vi "Teleop.vi"(10 "Match Info":T1={"Autonomous Elapsed Seconds"=0.0, "TeleOp Elapsed Seconds"=0.0, "Disabled Elapsed Seconds"=0.0, "Visited Autonomous"=FALSE, "Visited TeleOp"=FALSE, "Visited Disabled"=FALSE, "Autonomous Settings"={"Autonomous Style"=enum."Independent", "VI Refnum"=refnum}}, 11 "Call Context":T2) -> ()   [LabVIEW 2014]
doc: "This VI is called for each TeleOp packet received from the DS where the robot is not disabled. It is often used to read from the joysticks and update I/O or to update setpoints for timed control loops. It should complete and return within 20 milliseconds or it may miss DS packets."
uses:
  <vilib>/Rock Robotics/WPI/DriverStation/WPI_DriverStationDerivedRobotMode.ctl
  <vilib>/Rock Robotics/WPI/DriverStation/WPI_DriverStationMatch Info.ctl
  <vilib>/Rock Robotics/WPI/Solenoid/WPI_SolenoidValue.ctl
  <vilib>/Rock Robotics/WPI/Relay/WPI_RelayValue.ctl
  <vilib>/Rock Robotics/WPI/RobotDrive/WPI_RobotDriveGetSetRefNum.vi
  <vilib>/Rock Robotics/WPI/Joystick/WPI_JoystickGetSetRefNum.vi
  Robot Global Data.vi
  <vilib>/Rock Robotics/WPI/Solenoid/WPI_SolenoidSetEnum.vi
panel:
  in  "last switch":bool
  in  "toggle on/off internal":bool=TRUE
  out "toggle on/off":bool=TRUE
  out "Sample Slider 0":dbl(slide) scale=0.0..5.0
  out "Sample Boolean 1":bool
  out "Sample Boolean 0":bool
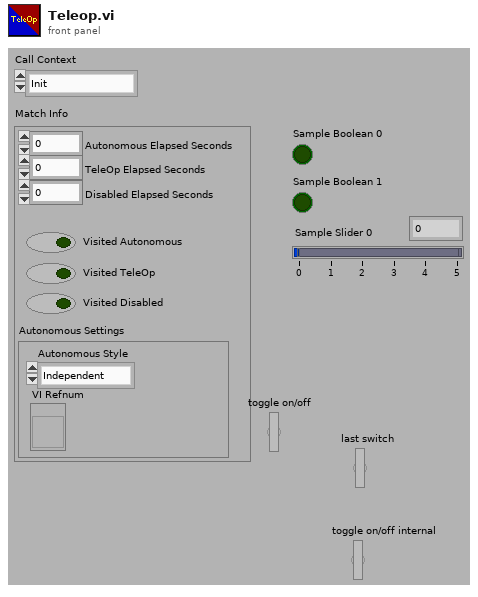
[diagram p1: front panel]
types:
  T1 = typedef "WPI_DriverStationMatch Info.ctl" = cluster{"Autonomous Elapsed Seconds":dbl, "TeleOp Elapsed Seconds":dbl, "Disabled Elapsed Seconds":dbl, "Visited Autonomous":bool, "Visited TeleOp":bool, "Visited Disabled":bool, "Autonomous Settings":cluster{"Autonomous Style":enum16{"Iterative", "Independent"}, "VI Refnum":refnum<vi>}}
  T2 = typedef "WPI_DriverStationDerivedRobotMode.ctl" = enum16{"Init", "Execute", "Stop"}
  T3 = typedef "WPI_RelayValue.ctl" = enum16{"Off", "On", "Forward", "Reverse"}
  T4 = typedef "WPI_SolenoidValue.ctl" = enum16{"Off", "On", "Forward", "Reverse"}
  T5 = typedef "WPI_RobotDriveDevRef.ctl" = cluster{"DevStatus":errorcluster, "Motors[]":T6[], "Square Inputs":bool, "Max Output":dbl}
  T6 = typedef "WPI_MotorControlDeviceRef.ctl" = cluster{"DeviceStatus":errorcluster, "Type":enum16{"PWM", "CAN"}, "PWM":cluster{"Digital Module":T7, "PWM Channel":T8, "DeadBand":T9}, "CAN":cluster{"Device Number":u8, "Control Mode":T10, "Semaphore":T11, "Max Vout":dbl}, "Invert":bool, "TransformRef":T12, "InvTransformRef":T12}
  T7 = typedef "FPGA_TypedefDigitalModule.ctl" = enum16{"Digital Module 1", "Digital Module 2"}
  T8 = typedef "FPGA_DIOPWMChannel.ctl" = enum8{"PWM 1", "PWM 2", "PWM 3", "PWM 4", "PWM 5", "PWM 6", "PWM 7", "PWM 8", "PWM 9", "PWM 10", "Invalid"}
  T9 = typedef "WPI_PWMDeadband.ctl" = cluster{"Name":string, "maxPositivePwm":i32, "minPositivePwm":i32, "centerPwm":i32, "maxNegativePwm":i32, "minNegativePwm":i32, "angularRange":u16}
  T10 = typedef "WPI_CANJaguar_ControlMode.ctl" = enum8{"Percent VBus", "Current", "Speed", "Position", "Voltage"}
  T11 = typedef "Semaphore RefNum" = refnum<k1>
  T12 = typedef "WPI_PWMTransform_ConPane.ctl" = refnum<vi>
  T13 = typedef "WPI_JoystickDevRef.ctl" = cluster{"Device":T14}
  T14 = typedef "WPI_JoystickDeviceEnum.ctl" = enum16{"USB 0", "USB 1", "USB 2", "USB 3", "USB 4", "USB 5"}
  T15 = typedef "WPI_RelayDevRef.ctl" = cluster{"DevStatus":errorcluster, "Relay Channel":T16, "Digital Module":T7, "Relay Direction":T17}
  T16 = typedef "FPGA_DIORelayChannel.ctl" = enum8{"Relay 1", "Relay 2", "Relay 3", "Relay 4", "Relay 5", "Relay 6", "Relay 7", "Relay 8", "Invalid"}
  T17 = typedef "WPI_RelayDirection.ctl" = enum16{"Both directions", "Forward only", "Reverse only"}
  T18 = typedef "WPI_SolenoidDevRef.ctl" = cluster{"DevStatus":errorcluster, "Solenoid Module":T19, "Forward Solenoid Channel":T20, "Reverse Solenoid Channel":T20}
  T19 = typedef "FPGA_TypedefSolenoidModule.ctl" = enum16{"Solenoid Module 1", "Solenoid Module 2"}
  T20 = typedef "WPI_SolenoidChannel.ctl" = enum8{"Solenoid 1", "Solenoid 2", "Solenoid 3", "Solenoid 4", "Solenoid 5", "Solenoid 6", "Solenoid 7", "Solenoid 8", "Invalid"}
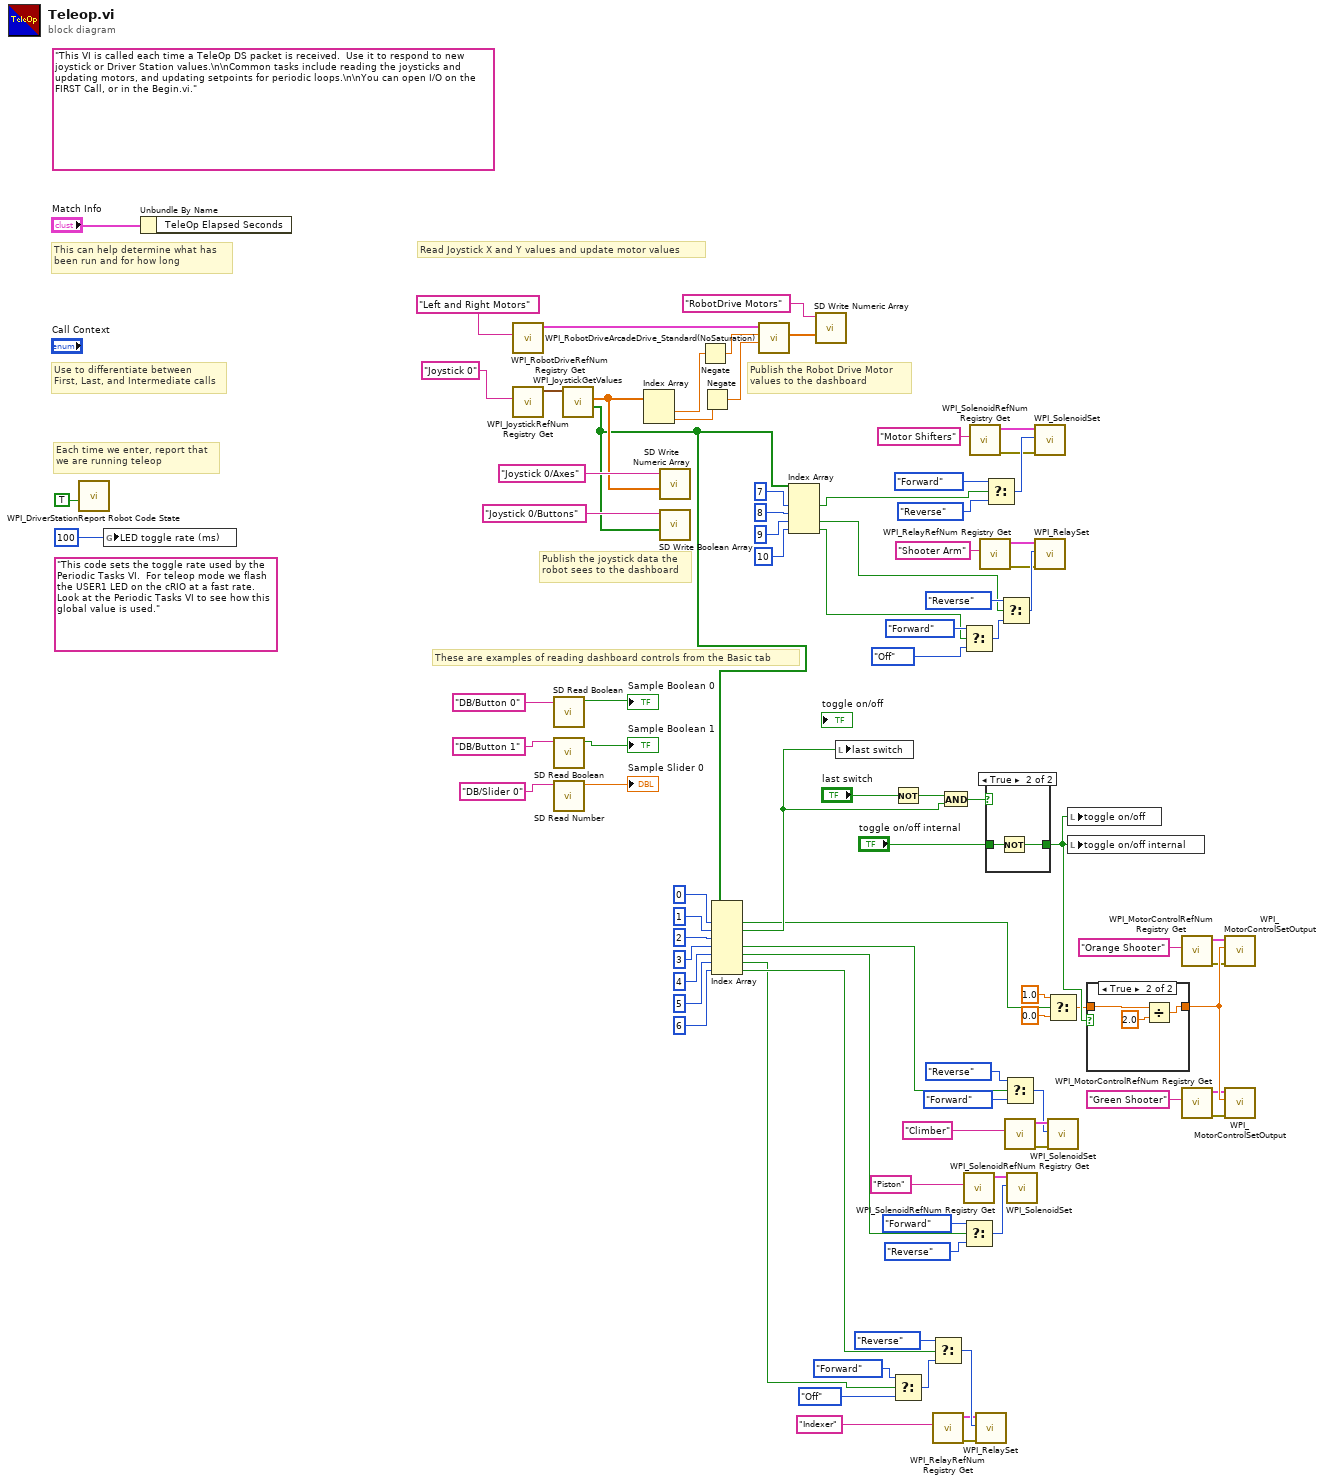
[diagram p0: block diagram]
diagram:
  (unwired) "This code sets the toggle rate used by the Periodic Tasks VI.  For teleop mode we flash the USER1 LED on the cRIO at a fast rate.  Look at the Periodic Tasks VI to see how this global value is used."
  (unwired) "This VI is called each time a TeleOp DS packet is received.  Use it to respond to new joystick or Driver Station values.\n\nCommon tasks include reading the joysticks and updating motors, and updating setpoints for periodic loops.\n\nYou can open I/O on the FIRST Call, or in the Begin.vi."
  # "These are examples of reading dashboard controls from the Basic tab"
  # "Publish the Robot Drive Motor\nvalues to the dashboard"
  # "Publish the joystick data the\nrobot sees to the dashboard"
  # "Each time we enter, report that\nwe are running teleop"
  # "Use to differentiate between\nFirst, Last, and Intermediate calls"
  # "This can help determine what has\nbeen run and for how long"
  # "Read Joystick X and Y values and update motor values"
  n1 = call <vilib>:"WPI_DriverStationReport Robot Code State.vi"("TeleOp"=TRUE ("Autonomous")) -> ()  [unwired: 10 in, 1 out]
  n2 = global write "Robot Global Data.vi" "LED toggle rate (ms)"(u32 100 ("LED ms toggle rate")) -> ()
  n3 = Unbundle By Name("Match Info") -> ()  [unwired: 1 out]
  n4 = call <vilib>:"WPI_RobotDriveRefNum Registry Get.vi"("refnum name"="Left and Right Motors") -> ("RobotDriveDevRef"=w89:T5)  [unwired: 1 in, 9 out]
  n5 = call <vilib>:"WPI_JoystickRefNum Registry Get.vi"("refnum name"="Joystick 0") -> ("JoystickDevRef"=w87:T13)  [unwired: 1 in, 9 out]
  n6 = call <vilib>:"SD Read Boolean.vi"("Name"="DB/Button 0" ("refnum name")) -> ("Boolean"=→"Sample Boolean 0":bool)  [unwired: 8 in, 2 out]
  n7 = call <vilib>:"SD Read Boolean.vi"("Name"="DB/Button 1" ("refnum name")) -> ("Boolean"=→"Sample Boolean 1":bool)  [unwired: 8 in, 2 out]
  n8 = call <vilib>:"SD Read Number.vi"("Name"="DB/Slider 0" ("refnum name")) -> ("Numeric"=→"Sample Slider 0":dbl)  [unwired: 8 in, 2 out]
  n9 = call <vilib>:"WPI_JoystickGetValues.vi"("JoystickDevRef"=w87) -> ("Buttons"=w37:bool[], "Axes"=w74:dbl[])  [unwired: 6 in, 3 out]
  n10 = Index Array(array=w74) -> (element #1=w3:dbl, element #2=w2:dbl)  [unwired: 2 in]
  n11 = call <vilib>:"SD Write Numeric Array.vi"("Numeric Array"=w74, "Name"="Joystick 0/Axes") -> ()  [unwired: 8 in, 2 out]
  n12 = call <vilib>:"SD Write Boolean Array.vi"("Boolean Array"=w37, "Name"="Joystick 0/Buttons") -> ()  [unwired: 8 in, 2 out]
  n13 = Negate(x=w3) -> (-x=w4:dbl)
  n14 = Negate(x=w2) -> (-x=w1:dbl)
  n15 = Index Array(array=w37, index #1=0 ("index"), index #2=1 ("index"), index #3=2 ("index"), index #4=3 ("index"), index #5=4 ("index"), index #6=5 ("index"), index #7=6 ("index")) -> (element #1=w28:bool, element #2=w29:bool, element #4=w8:bool, element #5=w7:bool, element #6=w5:bool, element #7=w6:bool)  [unwired: 1 out]
  n16 = call <vilib>:"WPI_RobotDriveArcadeDrive_Standard(NoSaturation).vi"("Y axis value"=w1, "X axis value"=w4, "RobotDriveDevRef"=w89) -> ("Motor Values"=w81:dbl[])  [unwired: 1 in, 7 out]
  n17 = Index Array(array=w37, index #1=7 ("index"), index #2=8 ("index"), index #3=9 ("index"), index #4=10 ("index")) -> (element #1=w55:bool, element #3=w54:bool, element #4=w53:bool)  [unwired: 1 out]
  n18 = call <vilib>:"SD Write Numeric Array.vi"("Numeric Array"=w81, "Name"="RobotDrive Motors") -> ()  [unwired: 8 in, 2 out]
  n19 = local write "last switch"(w29) -> ()
  n20 = Not(x="last switch") -> (.not. x?=w49:bool)
  n21 = Select(t=WPI_RelayValue."Forward" ("RelayValue"), s=w5, f=WPI_RelayValue."Off" ("RelayValue")) -> (s? t:f=w25:T3)
  n22 = Select(t=WPI_RelayValue."Reverse" ("RelayValue"), s=w6, f=w25) -> (s? t:f=w27:T3)
  n23 = call <vilib>:"WPI_RelayRefNum Registry Get.vi"("refnum name"="Indexer") -> ("error out"=w10:errorcluster, "RelayDevRef"=w9:T15)  [unwired: 9 in]
  n24 = And(x=w49, y=w29) -> (x .and. y?=w50:bool)
  n25 = Select(t=WPI_SolenoidValue."Forward" ("Value"), s=w53, f=WPI_RelayValue."Off" ("RelayValue")) -> (s? t:f=w72:T3)
  n26 = call <vilib>:"WPI_SolenoidRefNum Registry Get.vi"("refnum name"="Piston") -> ("SolenoidDevRef"=w12:T18)  [unwired: 9 in, 1 out]
  n27 = Select(t=WPI_SolenoidValue."Forward" ("Value"), s=w7, f=WPI_SolenoidValue."Reverse" ("Value")) -> (s? t:f=w16:T4)
  n28 = call <vilib>:"WPI_SolenoidRefNum Registry Get.vi"("refnum name"="Motor Shifters") -> ("error out"=w60:errorcluster, "SolenoidDevRef"=w61:T18)  [unwired: 9 in]
  n29 = call <vilib>:"WPI_RelaySet.vi"("error in (no error)"=w10, "RelayValue"=w27, "RelayDevRef"=w9) -> ()  [unwired: 7 in, 2 out]
  n30 = call <vilib>:"WPI_RelayRefNum Registry Get.vi"("refnum name"="Shooter Arm") -> ("error out"=w67:errorcluster, "RelayDevRef"=w68:T15)  [unwired: 9 in]
  n31 = Select(t=WPI_SolenoidValue."Forward" ("Value"), s=w55, f=WPI_SolenoidValue."Reverse" ("Value")) -> (s? t:f=w65:T4)
  n32 = case shown="True" w50 {
    tunnel: "toggle on/off internal" -> [w92 w94]
    tunnel: [w92 w93] -> w52
    frame False {
    }
    frame True {
      n33 = Not(x=w94) -> (.not. x?=w93:bool)
    }
  }
  n34 = Select(t=WPI_SolenoidValue."Reverse" ("Value"), s=w54, f=w72) -> (s? t:f=w73:T3)
  n35 = Select(t=WPI_SolenoidValue."Reverse" ("Value"), s=w8, f=WPI_SolenoidValue."Forward" ("Value")) -> (s? t:f=w17:T4)
  n36 = call <vilib>:"WPI_SolenoidRefNum Registry Get.vi"("refnum name"="Climber") -> ("error out"=w22:errorcluster, "SolenoidDevRef"=w21:T18)  [unwired: 9 in]
  n37 = call-poly <vilib>:"WPI_SolenoidSet.vi"("Value"=w16, "SolenoidDevRef"=w12) -> ()  [unwired: 8 in, 2 out]
  n38 = call-poly <vilib>:"WPI_SolenoidSet.vi"("error in (no error)"=w60, "Value"=w65, "SolenoidDevRef"=w61) -> ()  [unwired: 7 in, 2 out]
  n39 = call <vilib>:"WPI_RelaySet.vi"("error in (no error)"=w67, "RelayValue"=w73, "RelayDevRef"=w68) -> ()  [unwired: 7 in, 2 out]
  n40 = Select(t=1.0, s=w28, f=0.0) -> (s? t:f=w46:dbl)
  n41 = call-poly <vilib>:"WPI_SolenoidSet.vi"("error in (no error)"=w22, "Value"=w17, "SolenoidDevRef"=w21) -> ()  [unwired: 7 in, 2 out]
  n42 = local write "toggle on/off"(w52) -> ()
  n43 = local write "toggle on/off internal"(w52) -> ()
  n44 = case shown="True" w52 {
    tunnel: [w95 w96] -> w47
    tunnel: w46 -> [w95 w98]
    frame False {
    }
    frame True {
      n45 = Divide(x=w98, y=2.0) -> (x/y=w96:dbl)
    }
  }
  n46 = call <vilib>:"WPI_MotorControlRefNum Registry Get.vi"("refnum name"="Orange Shooter") -> ("error out"=w42:errorcluster, "MotorControlDevRef"=w43:T6)  [unwired: 9 in]
  n47 = call <vilib>:"WPI_MotorControlRefNum Registry Get.vi"("refnum name"="Green Shooter") -> ("error out"=w41:errorcluster, "MotorControlDevRef"=w40:T6)  [unwired: 9 in]
  n48 = call <vilib>:"WPI_MotorControlSetOutput.vi"("error in (no error)"=w42, "Output"=w47, "MotorControlDevRef"=w43) -> ()  [unwired: 6 in, 3 out]
  n49 = call <vilib>:"WPI_MotorControlSetOutput.vi"("error in (no error)"=w41, "Output"=w47, "MotorControlDevRef"=w40) -> ()  [unwired: 6 in, 3 out]
